vi "Drive Train Temps.vi"(8 "error in (no error)":errorcluster, 10 "Force Throttle?":bool, 11 "Tank Drive in":refnum<class "Tank Drive.lvclass">) -> (0 "error out":errorcluster, 2 "Drive Train Temperatures":T1={"Left Lead Temperature (C)"=nan, "Right Lead Temperature (C)"=nan, "Left Follows Temperatures (C)"=[], "Right Follows Temperatures (C)"=[]}, 3 "Tank Drive out":refnum<class "Tank Drive.lvclass">)   [LabVIEW 2019, in "Drive.lvlib" / "Tank Drive.lvclass"]
uses:
  Tank Drive.lvclass
  Controls/Drive Train Temperatures.ctl
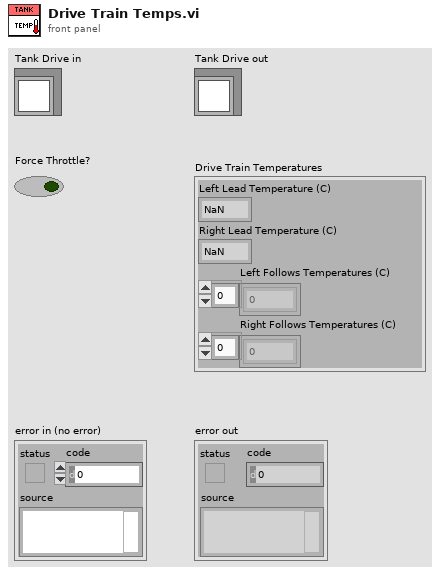
[diagram p1: front panel]
types:
  T1 = typedef "Drive.lvlib/Tank Drive.lvclass/Drive Train Temperatures.ctl" = cluster{"Left Lead Temperature (C)":dbl, "Right Lead Temperature (C)":dbl, "Left Follows Temperatures (C)":dbl[], "Right Follows Temperatures (C)":dbl[]}
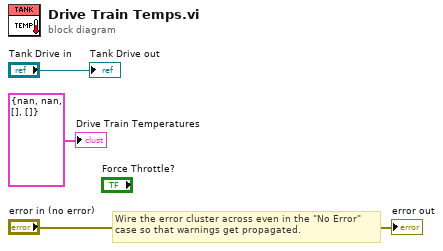
[diagram p0: block diagram]
diagram:
  # "Wire the error cluster across even in the \"No Error\"\ncase so that warnings get propagated."
  "error out" <- "error in (no error)"
  "Tank Drive out" <- "Tank Drive in"
  "Drive Train Temperatures" <- T1 {"Left Lead Temperature (C)"=nan, "Right Lead Temperature (C)"=nan, "Left Follows Temperatures (C)"=[], "Right Follows Temperatures (C)"=[]} ("input cluster")
